vi "DAQ_BASIC.vi"() -> ()   [LabVIEW 2018]
uses:
  <vilib>/DAQmx/configure/timing.llb/DAQmx Timing (Sample Clock).vi
  <vilib>/DAQmx/create/channels.llb/DAQmx Create Channel (AI-Voltage-Basic).vi
  <vilib>/DAQmx/read.llb/DAQmx Read (Analog 1D Wfm NChan NSamp).vi
  <vilib>/DAQmx/read.llb/DAQmx Read (Analog Wfm 1Chan 1Samp).vi
  <vilib>/DAQmx/read.llb/DAQmx Read (Analog Wfm 1Chan NSamp).vi
panel:
  out "웨이브폼 차트 4":waveform(dbl)(graph)
  out "웨이브폼 차트 3":waveform(dbl)(graph)
  in  "정지":bool
  in  "불리언":bool
  out "웨이브폼 차트":waveform(dbl)(graph)
  out "data":waveform(dbl)[](graph) caption="데이터"
  in  "stop":bool caption="정지"
  out "웨이브폼 차트 2":dynamicdata(graph)
  in  "stop (F) 2":bool caption="정지(F)"
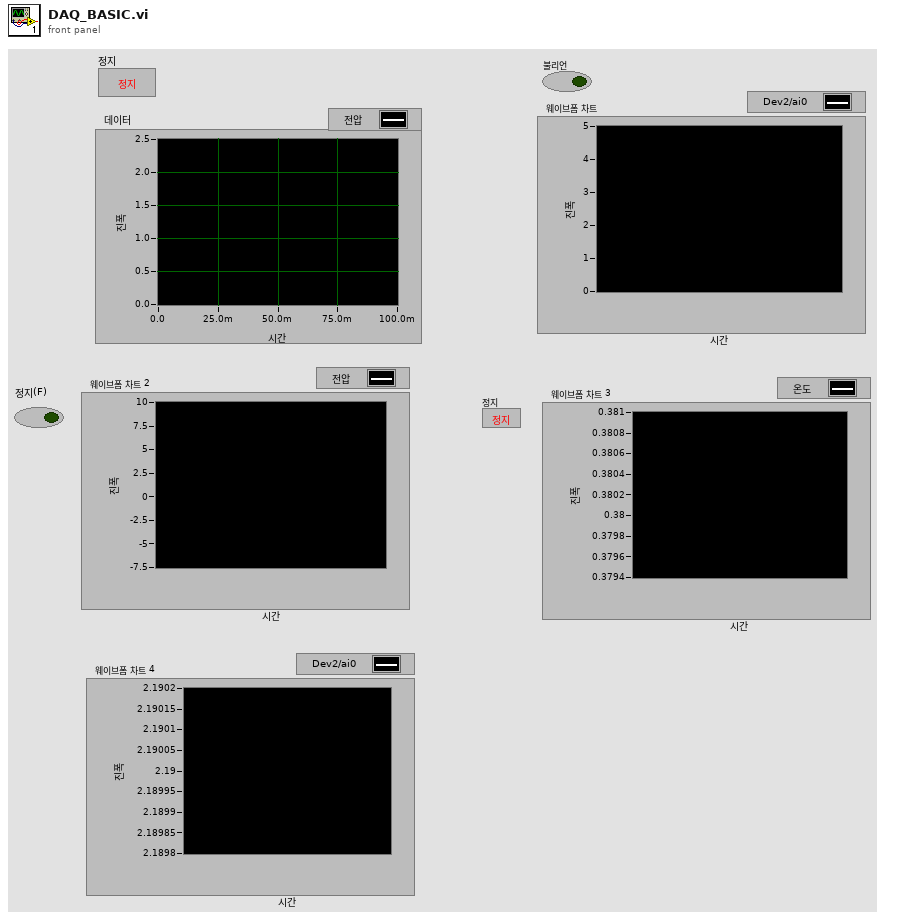
[diagram p1: front panel]
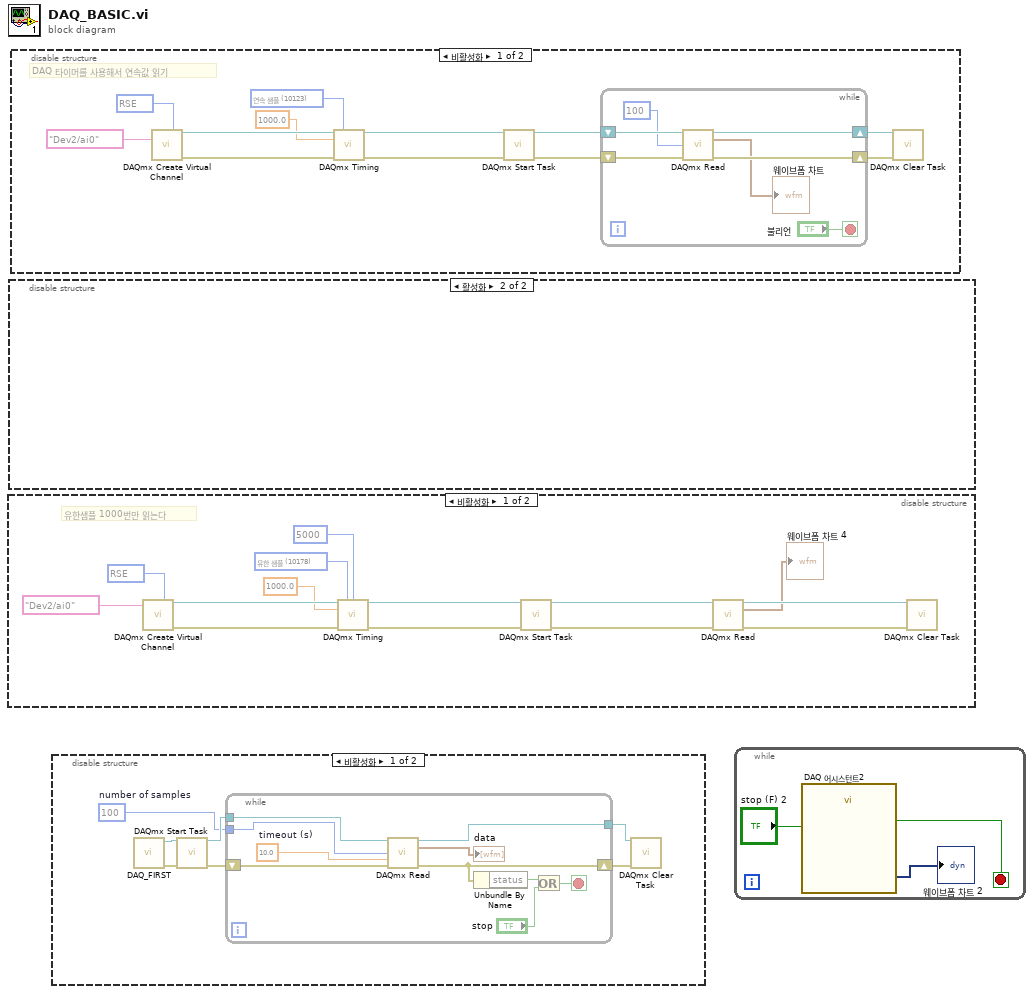
[diagram p0: block diagram]
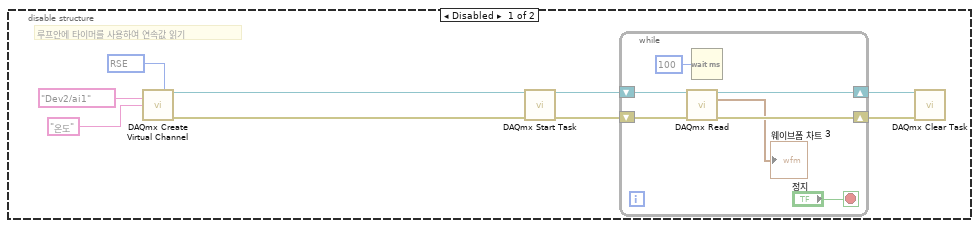
[diagram p3: hidden frame]
diagram:
  n1 = disable-structure shown="비활성화" {
    frame Disabled {
      w3 = 10178 items=["유한 샘플"=10178, "연속 샘플"=10123, "하드웨어 타이밍에 의한 단일 포인트"=12522] ("sample mode")
      w5 = 10083 items=["기본"=-1, "RSE"=10083, "NRSE"=10078, "차동"=10106, "유사 차동"=12529] ("input terminal configuration")
      # "유한샘플 1000번만 읽는다"
      n2 = call-poly <vilib>:"DAQmx Create Virtual Channel.vi"("input terminal configuration"=w5, "physical channels"=tag "Dev2/ai0") -> ("task out"=w14:refnum<k21>, "error out"=w13:errorcluster)  [unwired: 12 in]
      n3 = call-poly <vilib>:"DAQmx Timing.vi"("task/channels in"=w14, "sample mode"=w3, "samples per channel"=5000, "rate"=1000.0, "error in"=w13) -> ("task out"=w12:refnum<k21>, "error out"=w11:errorcluster)  [unwired: 9 in]
      n4 = call <vilib>:"DAQmx Start Task.vi"("task/channels in"=w12, "error in"=w11) -> ("task out"=w10:refnum<k21>, "error out"=w9:errorcluster)  [unwired: 12 in]
      n5 = call-poly <vilib>:"DAQmx Read.vi"("task/channels in"=w10, "error in"=w9) -> ("task out"=w8:refnum<k21>, "data"=→"웨이브폼 차트 4":waveform(dbl), "error out"=w7:errorcluster)  [unwired: 11 in]
      n6 = call <vilib>:"DAQmx Clear Task.vi"("task in"=w8, "error in"=w7) -> ()  [unwired: 13 in, 1 out]
    }
    frame Enabled {
    }
  }
  n7 = disable-structure shown="활성화" {
    frame Disabled {
      w18 = 10083 items=["기본"=-1, "RSE"=10083, "NRSE"=10078, "차동"=10106, "유사 차동"=12529] ("input terminal configuration")
      # "루프안에 타이머를 사용하여 연속값 읽기"
      n8 = call-poly <vilib>:"DAQmx Create Virtual Channel.vi"("input terminal configuration"=w18, "physical channels"=tag "Dev2/ai1", "name to assign"="온도") -> ("task out"=w16:refnum<k21>, "error out"=w15:errorcluster)  [unwired: 11 in]
      n9 = call <vilib>:"DAQmx Start Task.vi"("task/channels in"=w16, "error in"=w15) -> ("task out"=w23:refnum<k21>, "error out"=w22:errorcluster)  [unwired: 12 in]
      n10 = while {
        shift-right: [w28] -> w21
        shift-left: w23 -> [w30]
        shift-right: [w27] -> w20
        shift-left: w22 -> [w29]
        stop <- "정지" stop-if-true
        n11 = call-poly <vilib>:"DAQmx Read.vi"("task/channels in"=w30, "error in"=w29) -> ("task out"=w28:refnum<k21>, "data"=→"웨이브폼 차트 3":waveform(dbl), "error out"=w27:errorcluster)  [unwired: 11 in]
        n12 = Wait (ms)(milliseconds to wait=u32 100 ("대기 시간 (ms)")) -> ()  [unwired: 1 out]
      }
      n13 = call <vilib>:"DAQmx Clear Task.vi"("task in"=w21, "error in"=w20) -> ()  [unwired: 13 in, 1 out]
    }
    frame Enabled {
    }
  }
  n14 = disable-structure shown="비활성화" {
    frame Disabled {
      w31 = 10083 items=["기본"=-1, "RSE"=10083, "NRSE"=10078, "차동"=10106, "유사 차동"=12529] ("input terminal configuration")
      w32 = 10123 items=["유한 샘플"=10178, "연속 샘플"=10123, "하드웨어 타이밍에 의한 단일 포인트"=12522] ("sample mode")
      # "DAQ 타이머를 사용해서 연속값 읽기"
      n15 = call-poly <vilib>:"DAQmx Create Virtual Channel.vi"("input terminal configuration"=w31, "physical channels"=tag "Dev2/ai0") -> ("task out"=w42:refnum<k21>, "error out"=w41:errorcluster)  [unwired: 12 in]
      n16 = call-poly <vilib>:"DAQmx Timing.vi"("task/channels in"=w42, "sample mode"=w32, "rate"=1000.0, "error in"=w41) -> ("task out"=w40:refnum<k21>, "error out"=w39:errorcluster)  [unwired: 10 in]
      n17 = call <vilib>:"DAQmx Start Task.vi"("task/channels in"=w40, "error in"=w39) -> ("task out"=w38:refnum<k21>, "error out"=w37:errorcluster)  [unwired: 12 in]
      n18 = while {
        shift-right: [w47] -> w36
        shift-left: w38 -> [w49]
        shift-right: [w46] -> w35
        shift-left: w37 -> [w48]
        stop <- "불리언" stop-if-true
        n19 = call-poly <vilib>:"DAQmx Read.vi"("task/channels in"=w49, "number of samples per channel"=100, "error in"=w48) -> ("task out"=w47:refnum<k21>, "data"=→"웨이브폼 차트":waveform(dbl), "error out"=w46:errorcluster)  [unwired: 10 in]
      }
      n20 = call <vilib>:"DAQmx Clear Task.vi"("task in"=w36, "error in"=w35) -> ()  [unwired: 13 in, 1 out]
    }
    frame Enabled {
    }
  }
  n21 = disable-structure shown="비활성화" {
    frame Disabled {
      w54 = 100  # number of samples
      n22 = call "DAQ_FIRST.vi"() -> ("error out"=w50:errorcluster, "task out"=w51:refnum<k21>)  [unwired: 10 in]
      n23 = call <vilib>:"DAQmx Start Task.vi"("task/channels in"=w51, "error in"=w50) -> ("task out"=w56:refnum<k21>, "error out"=w55:errorcluster)  [unwired: 12 in]
      n24 = while "While 루프" {
        tunnel: w56 -> [w66]
        tunnel: w54 -> [w62]
        tunnel: [w63] -> w52
        shift-right: [w60] -> w53
        shift-left: w55 -> [w65]
        stop <- w59 stop-if-true
        w57 = 10.0  # timeout (s)
        n25 = call-poly <vilib>:"DAQmx Read.vi"("task/channels in"=w66, "number of samples per channel"=w62, "timeout"=w57, "error in"=w65) -> ("task out"=w63:refnum<k21>, "data"=→"data":waveform(dbl)[], "error out"=w60:errorcluster)  [unwired: 9 in]
        n26 = Unbundle By Name(w60) -> ("status"=w61:bool)
        n27 = Or(x=w61, y="stop") -> (x .or. y?=w59:bool)
      }
      n28 = call <vilib>:"DAQmx Clear Task.vi"("task in"=w52, "error in"=w53) -> ()  [unwired: 13 in, 1 out]
    }
    frame Enabled {
    }
  }
  n29 = while {
    stop <- w68 stop-if-true
    n30 = call "DAQ 어시스턴트2"("stop (F)"="stop (F) 2") -> ("data"=→"웨이브폼 차트 2":dynamicdata, "stopped"=w68:bool)  [unwired: 15 in, 2 out]
  }
